vi "Teleop_Out_Climb.vi"(8 "error in (no error)":errorcluster, 11 "Teleop Local Data Out":T1) -> (0 "error out":errorcluster)   [LabVIEW 2016]
uses:
  Typedefs/typedef_cluster_Teleop Local Data.ctl
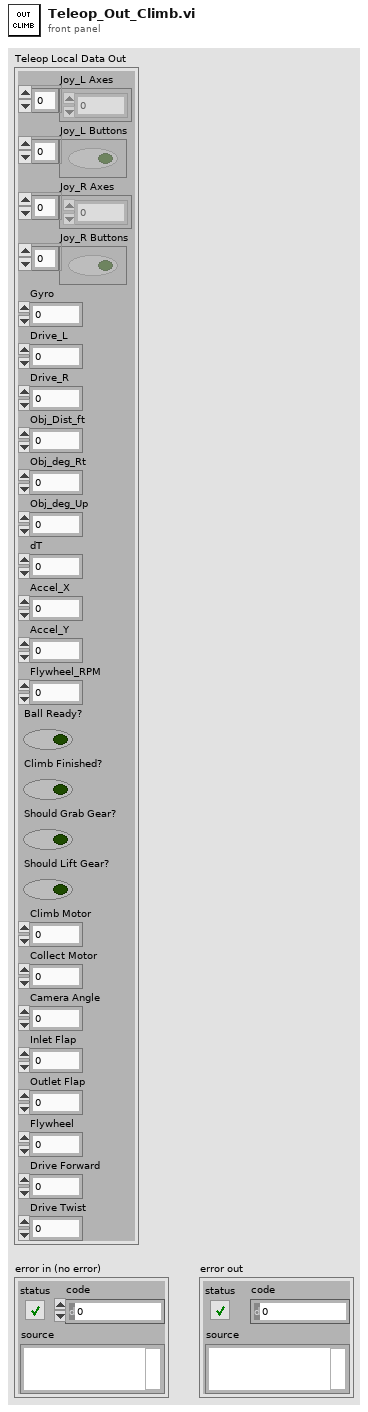
[diagram p1: front panel]
types:
  T1 = typedef "typedef_cluster_Teleop Local Data.ctl" = cluster{"Joy_L Axes":dbl[], "Joy_L Buttons":bool[], "Joy_R Axes":dbl[], "Joy_R Buttons":bool[], "Gyro":dbl, "Drive_L":i32, "Drive_R":i32, "Obj_Dist_ft":dbl, "Obj_deg_Rt":dbl, "Obj_deg_Up":dbl, "dT":dbl, "Accel_X":dbl, "Accel_Y":dbl, "Flywheel_RPM":dbl, "Ball Ready?":bool, "Climb Finished?":bool, "Should Grab Gear?":bool, "Should Lift Gear?":bool, "Climb Motor":dbl, "Collect Motor":dbl, "Camera Angle":dbl, "Inlet Flap":dbl, "Outlet Flap":dbl, "Flywheel":dbl, "Drive Forward":dbl, "Drive Twist":dbl}
  T2 = typedef "WPI_MotorControlDeviceRef.ctl" = cluster{"DeviceStatus":errorcluster, "Type":T3, "PWM":cluster{"PWM Channel":T4, "DeadBand":T5}, "CAN":cluster{"Device Number":u8, "SetOutput VI Ref":variant, "GetOutput VI Ref":variant, "Enable VI Ref":variant, "Disable VI Ref":variant, "Data":variant}, "Invert":bool}
  T3 = typedef "WPI_MotorControlType.ctl" = enum16{"PWM", "CAN"}
  T4 = typedef "FPGA_DIOPWMChannel.ctl" = enum8{"PWM 0", "PWM 1", "PWM 2", "PWM 3", "PWM 4", "PWM 5", "PWM 6", "PWM 7", "PWM 8", "PWM 9", "PWM MXP 0", "PWM MXP 1", "PWM MXP 2", "PWM MXP 3", "PWM MXP 4", "PWM MXP 5", "PWM MXP 6", "PWM MXP 7", "PWM MXP 8", "PWM MXP 9", "Invalid"}
  T5 = typedef "WPI_PWMDeadband.ctl" = cluster{"Name":string, "maxPositivePwm":i32, "minPositivePwm":i32, "centerPwm":i32, "maxNegativePwm":i32, "minNegativePwm":i32, "angularRange":u16}
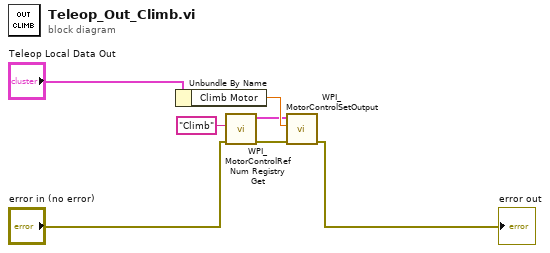
[diagram p0: block diagram]
diagram:
  n1 = Unbundle By Name("Teleop Local Data Out") -> ("Climb Motor"=w5:dbl)
  n2 = call <vilib>:"WPI_MotorControlRefNum Registry Get.vi"("error in (no error)"="error in (no error)", "refnum name"="Climb") -> ("error out"=w2:errorcluster, "MotorControlDevRef"=w3:T2)  [unwired: 8 in]
  n3 = call <vilib>:"WPI_MotorControlSetOutput.vi"("error in (no error)"=w2, "Output"=w5, "MotorControlDevRef"=w3) -> ("error out"=→"error out":errorcluster)  [unwired: 6 in, 2 out]
